vi "WriteData.vi"(0 "Message":string, 1 "File Prefix":string, 2 "base path":path) -> ()   [LabVIEW 2015]
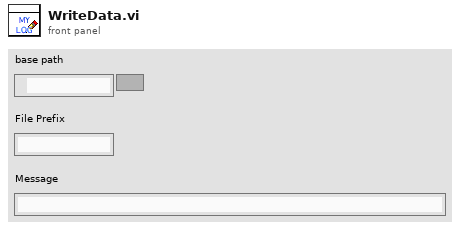
[diagram p1: front panel]
types:
  T1 = enum16{"open", "replace", "create", "open or create", "replace or create", "replace or create with confirmation"}
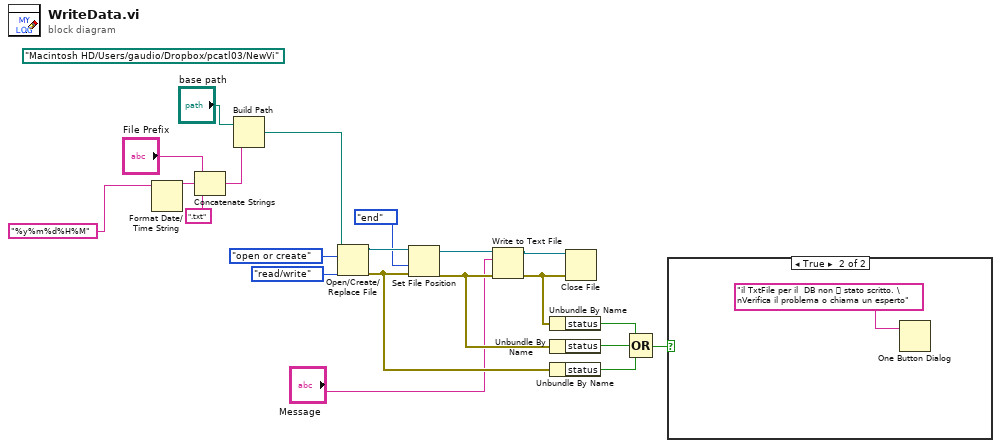
[diagram p0: block diagram]
diagram:
  (unwired) path "/Macintosh HD/Users/gaudio/Dropbox/pcatl03/NewVi" ("base path")
  n1 = Format Date/Time String(time format string (%c)="%y%m%d%H%M") -> (date/time string=w15:string)  [unwired: 2 in]
  n2 = Concatenate Strings("File Prefix", w15, ".txt" ("string")) -> (w13:string)
  n3 = Build Path(base path="base path", name or relative path=w13) -> (appended path=w12:path)
  n4 = Open/Create/Replace File(file path (use dialog)=w12, operation (0:open)=T1."open or create", access (0:read/write)=enum16{"read/write", "read-only", "write-only"}."read/write") -> (refnum out=w18:refnum<file>, error out=w10:errorcluster)  [unwired: 3 in, 1 out]
  n5 = Set File Position(refnum=w18, from (0:start)=enum16{"start", "end", "current"}."end", error in=w10) -> (refnum out=w17:refnum<file>, error out=w9:errorcluster)  [unwired: 1 in]
  n6 = Write to Text File(file (use dialog)=w17, text="Message", error in=w9) -> (refnum out=w20:refnum<file>, error out=w11:errorcluster)  [unwired: 1 in, 1 out]
  n7 = Unbundle By Name(w11) -> ("status"=w8:bool)
  n8 = Unbundle By Name(w9) -> ("status"=w7:bool)
  n9 = Unbundle By Name(w10) -> ("status"=w6:bool)
  n10 = Close File(refnum=w20, error in=w11) -> ()  [unwired: 2 out]
  n11 = Compound Arithmetic op=OR(w8, w7, w6) -> (w5:bool)
  n12 = case shown="True" w5 {
    frame False {
    }
    frame True {
      n13 = One Button Dialog(message="il TxtFile per il  DB non  stato scritto. \nVerifica il problema o chiama un esperto") -> ()  [unwired: 1 in, 1 out]
    }
  }
